vi "Initialize Workspace Control Refs.vi"(7 "T = PID":bool, 9 "State Variables in":T1={"UI.Chart.Refs"={"Chart"=refnum, "Manual Value"=refnum, "Manual Output"=refnum, "Revert"=refnum, "Apply"=refnum, "Setpoint"=refnum, "Autoscale X"=refnum, "Autoscale Y"=refnum, "Hold"=refnum, "Manual Control"=refnum}, "Addon.GUID"="", "Addon.Name"="", "Addon.Type"=enum."Industrial", "Data.UDPEngineQueue"=refnum, "Data.Found?"=FALSE, "Data.UDPChannels"=[], "Data.PreviousValues"=[], "Data.SlowChannels"=[], "Data.PendingChange?"=FALSE, "CachedData.UserEvent"=refnum, "CachedData.Data"={"Path"=""}, "Addon.Connected?"=FALSE, "NIVS.SysDefRoot"=refnum, "NIVS.Workspace"=refnum, "NIVS.UserEventRefs"={"Event Registration Refnum"=refnum, "SystemChangeEventRef"=refnum}, "NIVS.SystemStateRefs"={"CustDatRef"=refnum, "EvtRef"=refnum, "Target State User Event"=refnum}, "NIVS.LaunchRef"=refnum, "Setpoint Range"={"Min"=0.0, "Max"=0.0}, "Output Range"={"Min"=0.0, "Max"=0.0}, "UI.Device.Ref"=refnum}, 10 "Item.Data":T7, 11 "NIVS.Gateway IP Address":string) -> (0 "error out":errorcluster, 3 "State Variables out":T1={"UI.Chart.Refs"={"Chart"=refnum, "Manual Value"=refnum, "Manual Output"=refnum, "Revert"=refnum, "Apply"=refnum, "Setpoint"=refnum, "Autoscale X"=refnum, "Autoscale Y"=refnum, "Hold"=refnum, "Manual Control"=refnum}, "Addon.GUID"="", "Addon.Name"="", "Addon.Type"=enum."Industrial", "Data.UDPEngineQueue"=refnum, "Data.Found?"=FALSE, "Data.UDPChannels"=[], "Data.PreviousValues"=[], "Data.SlowChannels"=[], "Data.PendingChange?"=FALSE, "CachedData.UserEvent"=refnum, "CachedData.Data"={"Path"=""}, "Addon.Connected?"=FALSE, "NIVS.SysDefRoot"=refnum, "NIVS.Workspace"=refnum, "NIVS.UserEventRefs"={"Event Registration Refnum"=refnum, "SystemChangeEventRef"=refnum}, "NIVS.SystemStateRefs"={"CustDatRef"=refnum, "EvtRef"=refnum, "Target State User Event"=refnum}, "NIVS.LaunchRef"=refnum, "Setpoint Range"={"Min"=0.0, "Max"=0.0}, "Output Range"={"Min"=0.0, "Max"=0.0}, "UI.Device.Ref"=refnum})   [LabVIEW 2019, in "Control Workspace Object.lvlib"]
uses:
  Control Workspace Object.lvlib
  <vilib>/NI VeriStand/Execution/Workspace/NI_VS Workspace ExecutionAPI.lvlib
  Types/Workspace Object Cached Settings.ctl
  Types/UDP Streaming State.ctl
  Types/UDP Streaming Command Cluster.ctl
  Addon/Addon Shared/SubVIs/Constants.vi
  Addon/Addon Shared/Control Addon Shared.lvlib
  <vilib>/NI VeriStand/Display Template Support/DisplayTemplateSupport.llb/cluster_Graph Scale Settings.ctl
  <vilib>/NI VeriStand/Display Template Support/DisplayTemplateSupport.llb/cluster_Graph Plot Settings.ctl
  <vilib>/NI VeriStand/Display Template Support/DisplayTemplateSupport.llb/cluster_Screen Item Settings.ctl
  <vilib>/NI VeriStand/Display Template Support/DisplayTemplateSupport.llb/enum_Display Template Handler Minimal To Workspace.ctl
  NationalInstruments.VeriStand.SystemStorage
  NationalInstruments.VeriStand.ClientAPI
  <vilib>/NI VeriStand/Execution/Workspace/WorkspaceAPI.ctl
  <vilib>/NI VeriStand/Execution/Workspace/SystemStateRegEventRef.ctl
  <vilib>/NI VeriStand/Display Template Support/DisplayTemplateSupport.llb/enum_Display Template Handler Minimal To Widget Msg.ctl
  <vilib>/NI VeriStand/Execution/Workspace/SystemStateEventRef.ctl
  Types/Workspace Object State Variables.ctl
  <vilib>/NI VeriStand/Execution/Workspace/Target State.ctl
  <vilib>/NI VeriStand/Execution/Workspace/Target State Info.ctl
  Types/UI.Chart.Refs.ctl
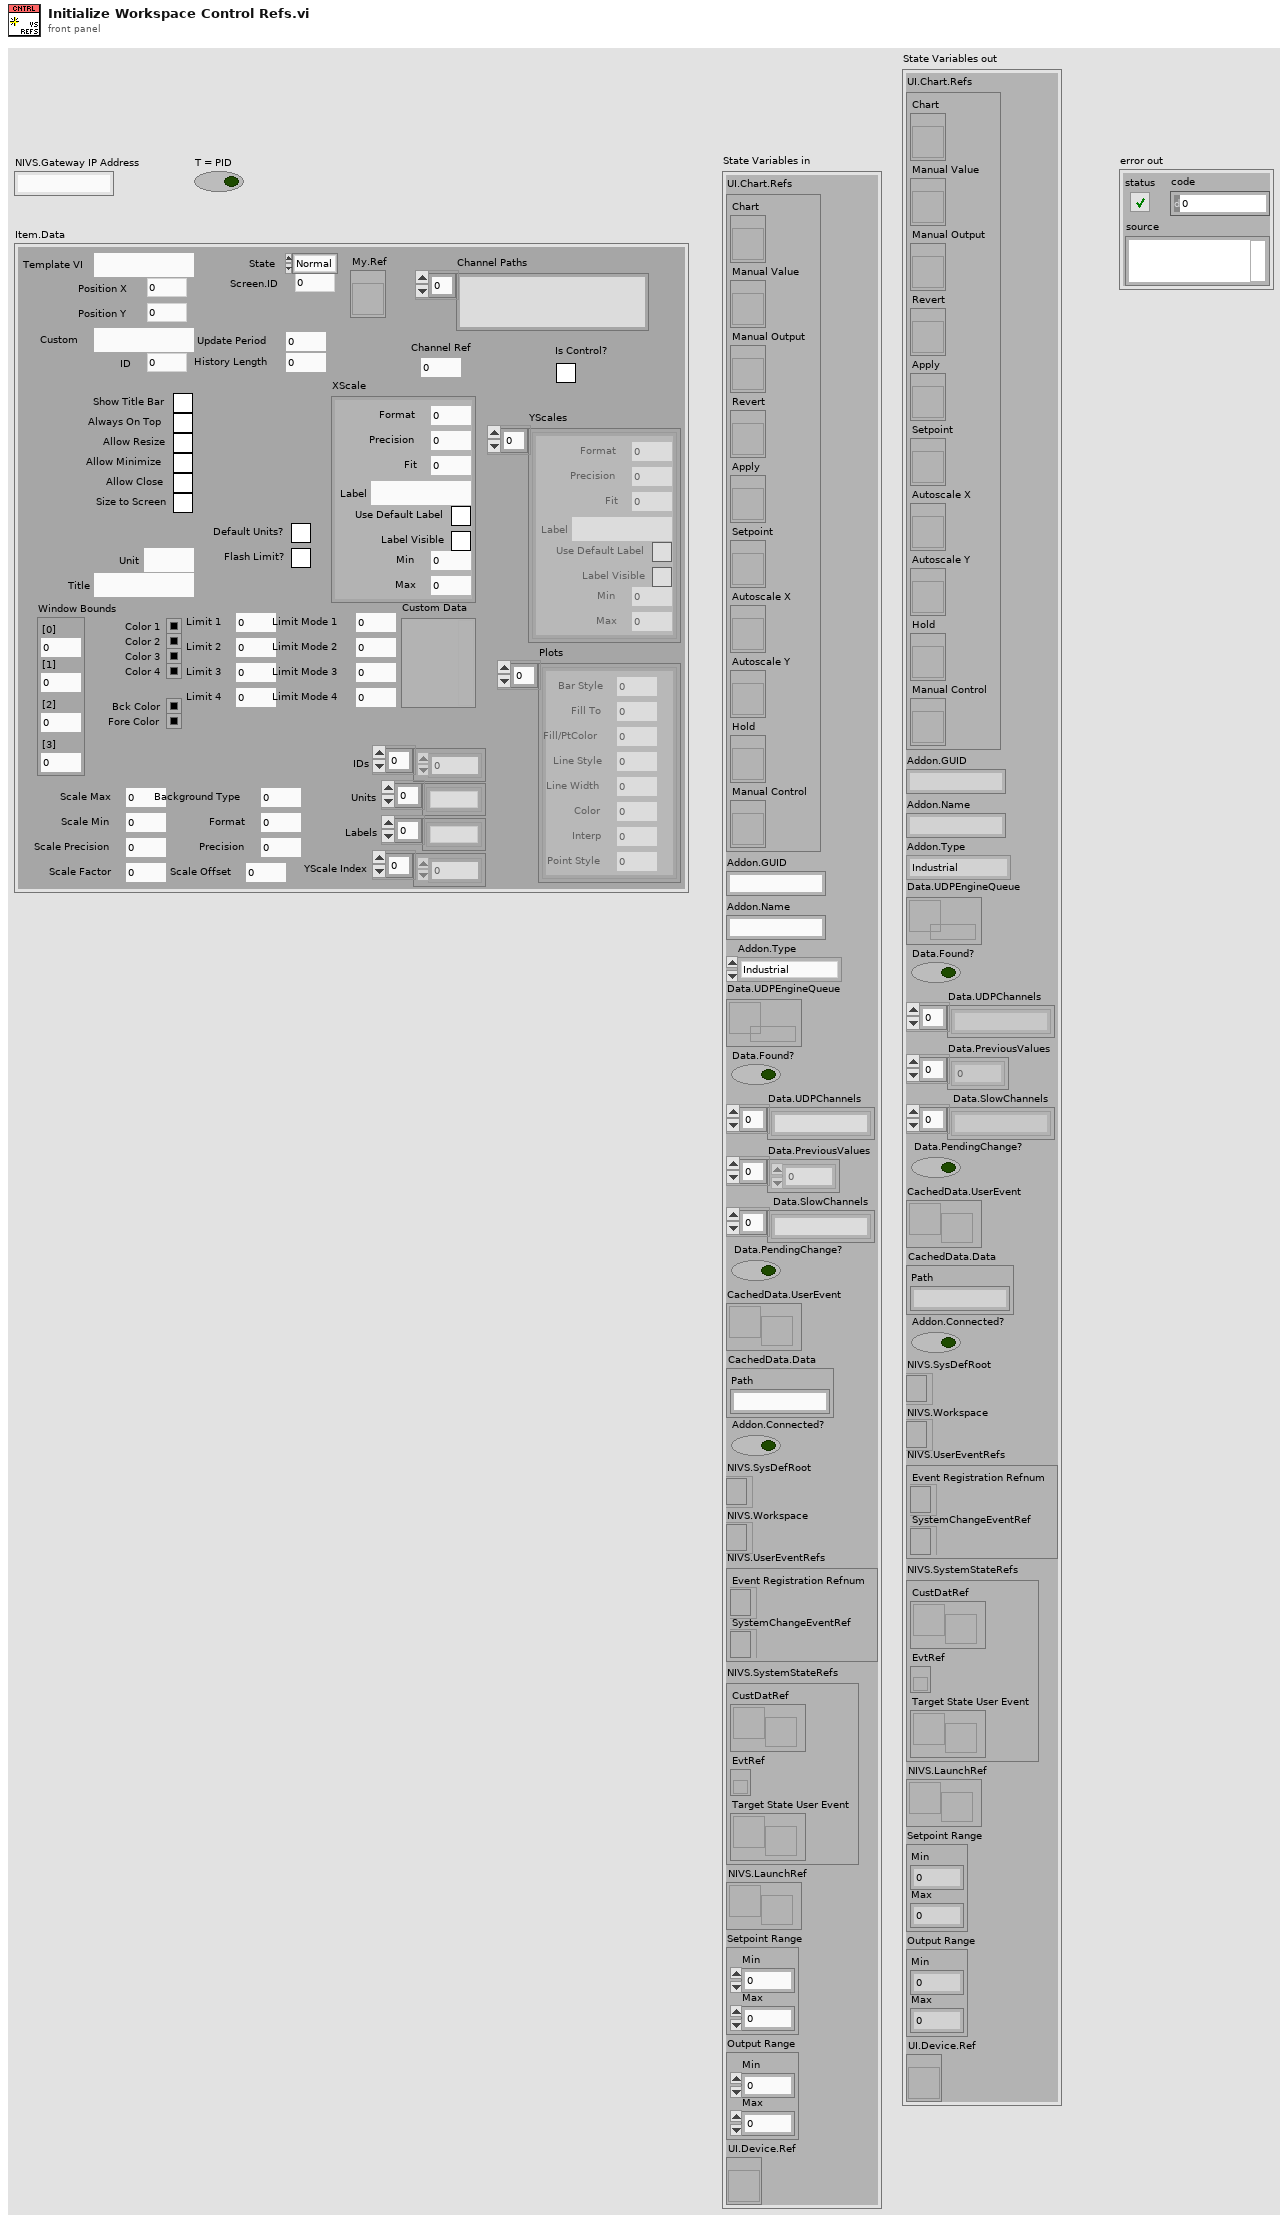
[diagram p1: front panel]
types:
  T1 = typedef "Control Workspace Object.lvlib/Workspace Object State Variables.ctl" = cluster{"UI.Chart.Refs":T2, "Addon.GUID":string, "Addon.Name":string, "Addon.Type":enum16{"PID", "Industrial"}, "Data.UDPEngineQueue":refnum<queue>, "Data.Found?":bool, "Data.UDPChannels":string[], "Data.PreviousValues":dbl[], "Data.SlowChannels":string[], "Data.PendingChange?":bool, "CachedData.UserEvent":refnum<user-event>, "CachedData.Data":T3, "Addon.Connected?":bool, "NIVS.SysDefRoot":refnum<k24>, "NIVS.Workspace":T4, "NIVS.UserEventRefs":cluster{"Event Registration Refnum":refnum<event-registration>, "SystemChangeEventRef":T5}, "NIVS.SystemStateRefs":T6, "NIVS.LaunchRef":refnum<user-event>, "Setpoint Range":cluster{"Min":dbl, "Max":dbl}, "Output Range":cluster{"Min":dbl, "Max":dbl}, "UI.Device.Ref":refnum<vi>}
  T2 = typedef "Control Workspace Object.lvlib/UI.Chart.Refs.ctl" = cluster{"Chart":refnum<vi>, "Manual Value":refnum<vi>, "Manual Output":refnum<vi>, "Revert":refnum<vi>, "Apply":refnum<vi>, "Setpoint":refnum<vi>, "Autoscale X":refnum<vi>, "Autoscale Y":refnum<vi>, "Hold":refnum<vi>, "Manual Control":refnum<vi>}
  T3 = typedef "Control Workspace Object.lvlib/Workspace Object Cached Settings.ctl" = cluster{"Path":string}
  T4 = typedef "NI_VS Workspace ExecutionAPI.lvlib/WorkspaceAPI.ctl" = refnum<k24>
  T5 = typedef "NI_VS Workspace ExecutionAPI.lvlib/SystemStateRegEventRef.ctl" = refnum<event-registration>
  T6 = typedef "NI_VS Workspace ExecutionAPI.lvlib/SystemStateEventRef.ctl" = cluster{"CustDatRef":refnum<user-event>, "EvtRef":refnum<k27>, "Target State User Event":refnum<user-event>}
  T7 = typedef "cluster_Screen Item Settings.ctl" = cluster{"Template VI":string, "Position X":i32, "Position Y":i32, "Custom":string, "Show Title Bar":bool, "ID":i32, "Always On Top":bool, "Allow Resize":bool, "Allow Minimize":bool, "Allow Close":bool, "Size to Screen":bool, "Screen.ID":i32, "State":enum16{"Normal", "New"}, "Title":string, "Window Bounds":cluster{"[0]":i16, "[1]":i16, "[2]":i16, "[3]":i16}, "Channel Ref":u64, "Unit":string, "Default Units?":bool, "Flash Limit?":bool, "Color 1":u32, "Color 2":u32, "Color 3":u32, "Color 4":u32, "Bck Color":u32, "Fore Color":u32, "Limit 1":dbl, "Limit 2":dbl, "Limit 3":dbl, "Limit 4":dbl, "Limit Mode 1":i32, "Limit Mode 2":i32, "Limit Mode 3":i32, "Limit Mode 4":i32, "Scale Precision":i32, "Scale Min":dbl, "Scale Max":dbl, "Format":i32, "Precision":i32, "Background Type":i32, "IDs":i32[], "Units":string[], "Labels":string[], "Scale Factor":dbl, "Scale Offset":dbl, "YScale Index":u32[], "XScale":T8, "YScales":T8[], "Plots":T9[], "Update Period":dbl, "History Length":dbl, "My.Ref":refnum<vi>, "Is Control?":bool, "Channel Paths":string[], "Custom Data":variant}
  T8 = typedef "cluster_Graph Scale Settings.ctl" = cluster{"Format":u8, "Precision":u8, "Fit":u8, "Label":string, "Use Default Label":bool, "Label Visible":bool, "Min":dbl, "Max":dbl}
  T9 = typedef "cluster_Graph Plot Settings.ctl" = cluster{"Bar Style":u8, "Fill To":i16, "Fill/PtColor":u32, "Line Style":u8, "Line Width":u8, "Color":u32, "Interp":u8, "Point Style":u8}
  T10 = typedef "Control Workspace Object.lvlib/UDP Streaming Command Cluster.ctl" = cluster{"Action":T11, "Channels":string[]}
  T11 = typedef "Control Workspace Object.lvlib/UDP Streaming State.ctl" = enum8{"Idle", "Start Acq", "Run", "Stop Acq", "Exit"}
  T12 = cluster{"Event Registration Refnum":refnum<event-registration>, "SystemChangeEventRef":T5}
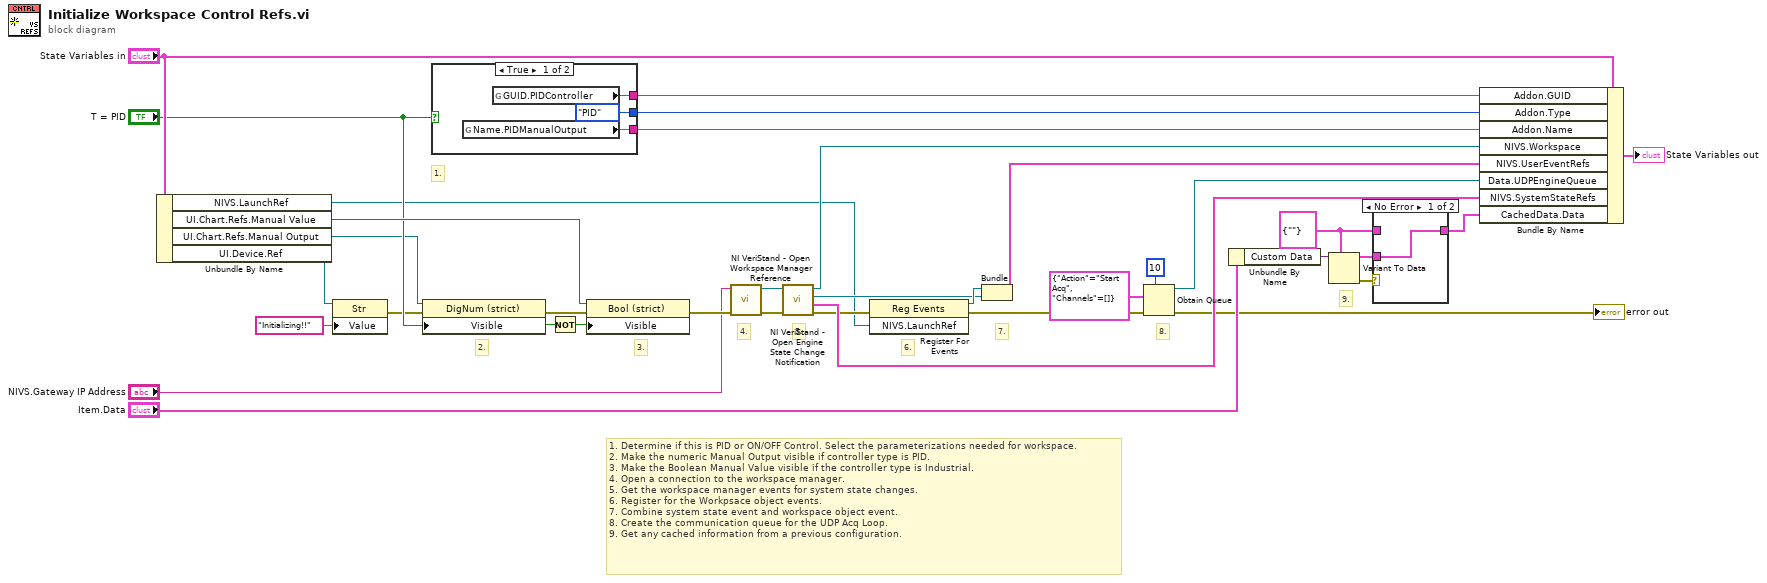
[diagram p0: block diagram]
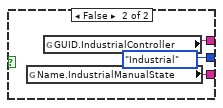
[diagram p2: hidden frame]
diagram:
  w18 = T3 {"Path"=""}
  # "1. Determine if this is PID or ON/OFF Control. Select the parameterizations needed for workspace.\n2. Make the numeric Manual Output visible if controller type is PID.\n3. Make the Boolean Manual Value visible if the controller type is Industrial.\n4. Open a connection to the workspace manager.\n5. Get the workspace manager events for system state changes.\n6. Register for the Workpsace object events.\n7. Combine system state event and workspace object event.\n8. Create the communication queue for the UDP Acq Loop.\n9. Get any cached information from a previous configuration."
  # "9."
  # "8."
  # "7."
  # "6."
  # "5."
  # "4."
  # "3."
  # "2."
  # "1."
  n1 = Unbundle By Name("State Variables in") -> ("NIVS.LaunchRef"=w6:refnum<user-event>, "UI.Chart.Refs.Manual Value"=w30:refnum<vi>, "UI.Chart.Refs.Manual Output"=w28:refnum<vi>, "UI.Device.Ref"=w2:refnum<vi>)
  n2 = property class="Str"(reference=w2, "Value"="Initializing!!") -> (error out=w3:errorcluster)  [unwired: 1 in, 1 out]
  n3 = property class="DigNum (strict)"(reference=w28, error in=w3, "Visible"="T = PID") -> (error out=w32:errorcluster)  [unwired: 1 out]
  n4 = case shown="True" "T = PID" {
    tunnel: [w38 w41] -> w23
    tunnel: [w36 w40] -> w21
    tunnel: [enum16{"PID", "Industrial"}."PID" ("Type") enum16{"PID", "Industrial"}."Industrial" ("Type")] -> w22
    frame True {
      n5 = global read "Constants.vi" "Name.PIDManualOutput"() -> (w36:string)
      n6 = global read "Constants.vi" "GUID.PIDController"() -> (w38:string)
    }
    frame False {
      n7 = global read "Constants.vi" "Name.IndustrialManualState"() -> (w40:string)
      n8 = global read "Constants.vi" "GUID.IndustrialController"() -> (w41:string)
    }
  }
  n9 = Not(x="T = PID") -> (.not. x?=w31:bool)
  n10 = property class="Bool (strict)"(reference=w30, error in=w32, "Visible"=w31) -> (error out=w33:errorcluster)  [unwired: 1 out]
  n11 = call <vilib>:"NI VeriStand - Open Workspace Manager Reference.vi"("error in (no error)"=w33, "Gateway IP Address (\"\": localhost)"="NIVS.Gateway IP Address") -> ("error out"=w12:errorcluster, "WorkspaceManager"=w26:T4)  [unwired: 8 in]
  n12 = call <vilib>:"NI VeriStand - Open Engine State Change Notification.vi"("error in (no error)"=w12, "WorkspaceManager in"=w26) -> ("error out"=w8:errorcluster, "SystemStateRefs"=w25:T6, "SystemChangeEventRef"=w13:T5, "WorkspaceManager out"=w9:T4)  [unwired: 6 in]
  n13 = register-events(error in=w8, w6) -> (reference out=w14:refnum<event-registration>, error out=w7:errorcluster)  [unwired: 1 in]
  n14 = Bundle("Event Registration Refnum"=w14, "SystemChangeEventRef"=w13) -> (w24:T12)  [unwired: 1 in]
  n15 = Obtain Queue(max queue size (-1, unlimited)=10, element data type=T10 {"Action"=enum."Start Acq", "Channels"=[]}, error in (no error)=w7) -> (queue out=w5:refnum<queue>, error out=→"error out":errorcluster)  [unwired: 2 in, 1 out]
  n16 = Unbundle By Name("Item.Data") -> ("Custom Data"=w15:variant)
  n17 = Variant To Data(type=w18, Variant=w15) -> (data=w17:T3, error out=w16:errorcluster)  [unwired: 1 in]
  n18 = case shown="No Error" w16 {
    tunnel: w17 -> [w42 _]
    tunnel: [w42 w43] -> w4
    tunnel: w18 -> [_ w43]
    frame No Error {
    }
    frame Error {
    }
  }
  n19 = Bundle By Name(cluster="State Variables in", "Addon.GUID"=w23, "Addon.Type"=w22, "Addon.Name"=w21, "NIVS.Workspace"=w9, "NIVS.UserEventRefs"=w24, "Data.UDPEngineQueue"=w5, "NIVS.SystemStateRefs"=w25, "CachedData.Data"=w4) -> (→"State Variables out":T1)
